vi "digit to color converter.vi"(4 "Digit select":T1) -> (1 "Digit color":u32(colorbox))   [LabVIEW 2018]
uses:
  digit--control.ctl
  Resistor Band Colors/Resistor Band Colors.lvlib
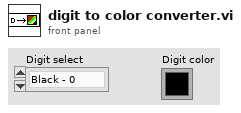
[diagram p1: front panel]
types:
  T1 = typedef "digit--control.ctl" = enum16{"Black - 0", "Brown - 1", "Red - 2", "Orange - 3", "Yellow - 4", "Green - 5", "Blue - 6", "Violet - 7", "Grey - 8", "White - 9"}
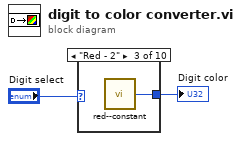
[diagram p0: block diagram]
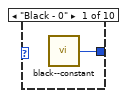
[diagram p2: hidden frame]
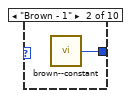
[diagram p3: hidden frame]
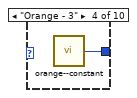
[diagram p4: hidden frame]
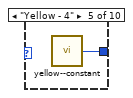
[diagram p5: hidden frame]
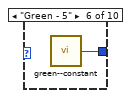
[diagram p6: hidden frame]
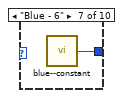
[diagram p7: hidden frame]
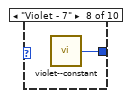
[diagram p8: hidden frame]
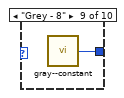
[diagram p9: hidden frame]
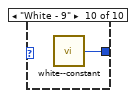
[diagram p10: hidden frame]
diagram:
  n1 = case shown="\"Red - 2\"" "Digit select" {
    tunnel: [w3 w4 w5 w6 w7 w8 w9 w10 w11 w12] -> w1
    frame "Black - 0" {
      n2 = call "black--constant.vi"() -> ("Black"=w3:u32)  [unwired: 5 in]
    }
    frame "Brown - 1" {
      n3 = call "brown--constant.vi"() -> ("Brown"=w4:u32)  [unwired: 5 in]
    }
    frame "Red - 2" {
      n4 = call "red--constant.vi"() -> ("Red"=w5:u32)  [unwired: 5 in]
    }
    frame "Orange - 3" {
      n5 = call "orange--constant.vi"() -> ("Orange"=w6:u32)  [unwired: 5 in]
    }
    frame "Yellow - 4" {
      n6 = call "yellow--constant.vi"() -> ("Yellow"=w7:u32)  [unwired: 5 in]
    }
    frame "Green - 5" {
      n7 = call "green--constant.vi"() -> ("Green"=w8:u32)  [unwired: 5 in]
    }
    frame "Blue - 6" {
      n8 = call "blue--constant.vi"() -> ("Blue"=w9:u32)  [unwired: 5 in]
    }
    frame "Violet - 7" {
      n9 = call "violet--constant.vi"() -> ("Violet"=w10:u32)  [unwired: 5 in]
    }
    frame "Grey - 8" {
      n10 = call "gray--constant.vi"() -> ("Gray"=w11:u32)  [unwired: 5 in]
    }
    frame "White - 9" {
      n11 = call "white--constant.vi"() -> ("White"=w12:u32)  [unwired: 5 in]
    }
  }
  "Digit color" <- w1
